vi "PTSequencer.update DIM subscriptions.vi"(0 "i ref in":refnum<vi>, 3 "ms timeout (10000)":i32=10000, 5 "error in":errorcluster) -> (14 "i ref out":refnum<vi>, 17 "timed out":bool, 19 "error out":errorcluster)   [LabVIEW 2014, in "PTSequencer.lvlib"]
uses:
  PTSequencer.lvlib
  CSCore/BaseProcess/BaseProcess.lvlib
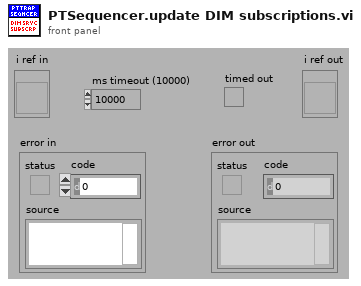
[diagram p1: front panel]
types:
  T1 = typedef "PTSequencer.lvlib/PTSequencer.i attribute.ctl" = cluster{"subsequence":bool, "mode":T2, "i step":i32, "nofLoops":i32, "i loop":i32, "Running":bool, "Paused":bool, "step done":bool, "loop done":bool, "seq done":bool, "DIM IDs":cluster{"step done":i32, "loop done":i32, "seq done":i32, "i step":i32, "i loop":i32}, "use stop conditions":bool, "stop conditions":T3[], "Step List":T5[], "DIM subsriptions":string[], "stop cond indexes":i32[], "step cond indexes":cluster{"step condition IDs":cluster{"step ID":i32, "condition ID":i32}[]}[], "Delay Start Time":timestamp, "status":string, "stopping":bool}
  T2 = typedef "PTSequencer.lvlib/PTSequencer.mode.ctl" = enum16{"single", "loop", "for loop"}
  T3 = typedef "PTSequencer.lvlib/PTSequencer.DIM service condition.ctl" = cluster{"DIM service":string, "descr":string, "nomValue":T4, "actValue":T4, "matched":bool, "DIM Status":cluster{"no link":bool, "quality":i32, "Time Stamp":timestamp}}
  T4 = typedef "CoreDefs.rawDataType.ctl" = i8[]
  T5 = typedef "PTSequencer.lvlib/PTSequencer.step.ctl" = cluster{"description":string, "object parameters":cluster{"object":string, "selector":string, "descriptor":string, "data":T4, "subsequence":bool, "call mode":enum16{"Simple DIM", "Synchronous"}, "data in":T4}, "result action":cluster{"check":bool, "passed":enum16{"Next", "Previous", "Repeat", "Jump"}, "failed":enum16{"Next", "Previous", "Repeat", "Jump"}, "jumpID_passed":i32, "jumpID_failed":i32}, "conditions":T3[], "fulfilled ":bool, "use delay":bool, "delay time (s)":dbl, "ID":i32}
  T6 = typedef "BaseProcess.lvlib/BaseProcess.event definition.ctl" = cluster{"CAEEvtDef":T7, "Data Descriptor":T8}
  T7 = typedef "CAEObj.lvlib/CAEObj.event definition.ctl" = cluster{"URL":string, "enable":bool, "ignoreResID":bool}
  T8 = typedef "BaseProcess.lvlib/BaseProcess.descriptor string definition.ctl" = string
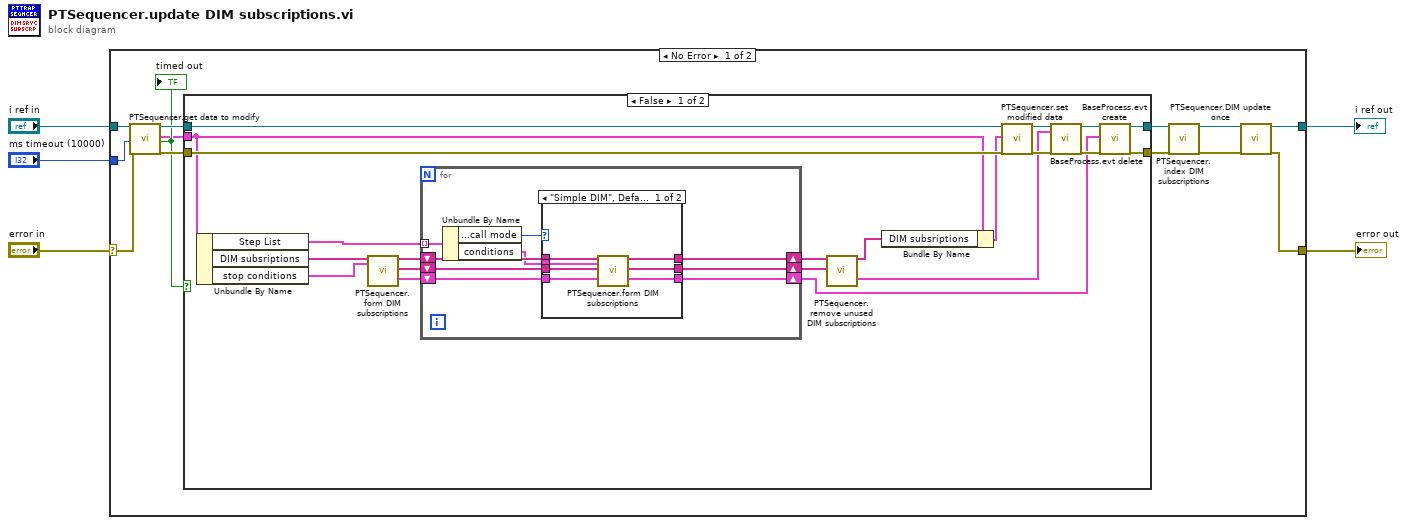
[diagram p0: block diagram]
diagram:
  n1 = case shown="No Error" "error in" {
    selector: "error in" -> [w18 w61]
    tunnel: "i ref in" -> [w15 w62]
    tunnel: [w7 w62] -> w4
    tunnel: [w6 w61] -> w3
    tunnel: "ms timeout (10000)" -> [w12 _]
    frame No Error {
      n2 = call "PTSequencer.get data to modify.vi"("i ref in"=w15, "ms timeout (10000)"=w12, "error in (no error)"=w18) -> ("i ref out"=w16:refnum<vi>, "i attribute"=w13:T1, "timed out"=w14:bool, "error out"=w17:errorcluster)  [unwired: 13 in]
      "timed out" <- w14
      n3 = case shown="False" w14 {
        tunnel: [w39 w60] -> w11
        tunnel: w17 -> [w37 w59]
        tunnel: w16 -> [w38 w60]
        tunnel: w13 -> [w31 _]
        tunnel: [w20 w59] -> w10
        frame False {
          n4 = Unbundle By Name(w31) -> ("Step List"=w29:T5[], "DIM subsriptions"=w30:string[], "stop conditions"=w25:T3[])
          n5 = call "PTSequencer.form DIM subscriptions.vi"("DIM subsriptions"=w30, "conditions"=w25) -> ("DIM subsriptions out"=w28:string[], "used subsriptions out"=w27:string[], "trendmsgs out"=w26:T6[])  [unwired: 15 in]
          n6 = for {
            tunnel: w29 -> [w40] mode=indexing
            shift-right: [w45] -> w24
            shift-left: w28 -> [w48]
            shift-right: [w41] -> w23
            shift-left: w27 -> [w44]
            shift-right: [w42] -> w21
            shift-left: w26 -> [w43]
            n7 = Unbundle By Name(w40) -> ("object parameters.call mode"=w46:enum16{"Simple DIM", "Synchronous"}, "conditions"=w47:T3[])
            n8 = case shown="\"Simple DIM\", Default" w46 {
              tunnel: w48 -> [w55 w58]
              tunnel: w47 -> [w49 _]
              tunnel: [w54 w58] -> w45
              tunnel: w44 -> [w53 w57]
              tunnel: w43 -> [w52 w56]
              tunnel: [w51 w56] -> w42
              tunnel: [w50 w57] -> w41
              frame "Simple DIM", Default {
                n9 = call "PTSequencer.form DIM subscriptions.vi"("DIM subsriptions"=w55, "conditions"=w49, "used subsriptions in"=w53, "trendmsgs in"=w52) -> ("DIM subsriptions out"=w54:string[], "used subsriptions out"=w50:string[], "trendmsgs out"=w51:T6[])  [unwired: 13 in]
              }
              frame "Synchronous" {
              }
            }
          }
          n10 = call "PTSequencer.remove unused DIM subscriptions.vi"("DIM subsriptions"=w24, "Used subsriptions"=w23) -> ("DIM subsriptions out"=w19:string[], "msgs to remove"=w22:T6[])  [unwired: 16 in]
          n11 = Bundle By Name(cluster=w31, "DIM subsriptions"=w19) -> (w36:T1)
          n12 = call "PTSequencer.set modified data.vi"("i ref in"=w38, "CLASS.i attribute"=w36, "error in (no error)"=w37) -> ("i ref out"=w35:refnum<vi>, "error out"=w33:errorcluster)  [unwired: 15 in]
          n13 = call "BaseProcess.evt delete.vi"("i ref in"=w35, "events"=w22, "error in (no error)"=w33) -> ("i ref out"=w34:refnum<vi>, "error out"=w32:errorcluster)  [unwired: 13 in, 2 out]
          n14 = call "BaseProcess.evt create.vi"("i ref in"=w34, "newEvents"=w21, "error in (no error)"=w32) -> ("i ref out"=w39:refnum<vi>, "error out"=w20:errorcluster)  [unwired: 13 in, 2 out]
        }
        frame True {
        }
      }
      n15 = call "PTSequencer.index DIM subscriptions.vi"("i ref in"=w11, "error in"=w10) -> ("i ref out"=w9:refnum<vi>, "error out"=w8:errorcluster)  [unwired: 15 in, 1 out]
      n16 = call "PTSequencer.DIM update once.vi"("i ref in"=w9, "error in"=w8) -> ("i ref out"=w7:refnum<vi>, "error out"=w6:errorcluster)  [unwired: 15 in, 1 out]
    }
    frame Error {
    }
  }
  "i ref out" <- w4
  "error out" <- w3
